vi "Fetch.vi"(8 "error in (no error)":errorcluster, 10 "Message in":refnum<class "FetchMessage.lvclass">, 11 "BMC in":refnum<class "BMC.lvclass">) -> (0 "error out":errorcluster, 3 "BMC out":refnum<class "BMC.lvclass">)   [LabVIEW 2012, in "BMC.lvclass"]
doc: "The fetch method processes the command 'fetch'. \n\nThe command 'fetch' is used for receiving various forms of data."
uses:
  BMC.lvclass
  <vilib>/Distrio/Murmex/FetchMessage/FetchMessage.lvclass
  <vilib>/Distrio/Murmex/Murmex/Murmex.lvclass
  BMC.lvclass/BMC.ctl
panel:
  out "actuator":dbl
  out "1x160 voltage array":dbl[](array[numeric])
  # "This method is called when the FETCH\ntrigger is sent. \n\nOverride this method when your component needs to\nrespond to this trigger. \n\nCall parent for proper implementation"
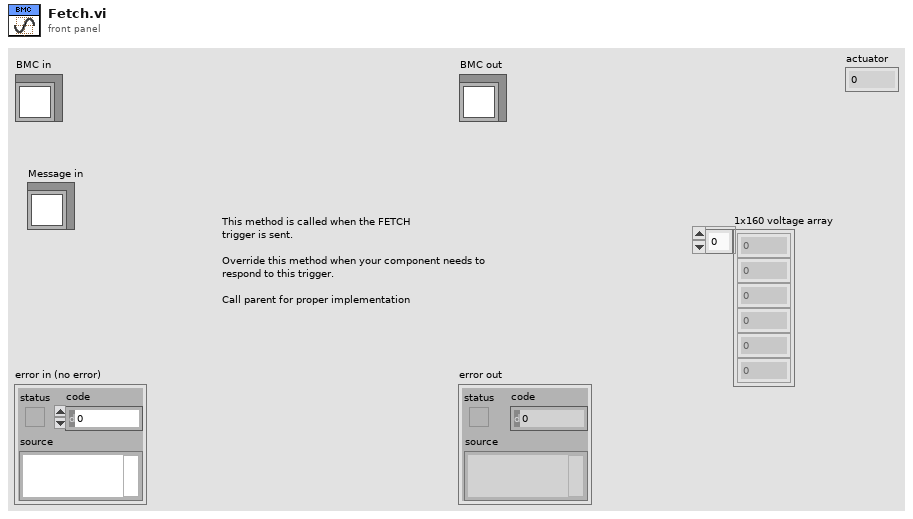
[diagram p1: front panel]
types:
  T1 = typedef "Murmex.lvlib/FetchMessage.lvclass/Channel data cluster.ctl" = cluster{"channel id":i32, "data UInt8":u8[], "data type":T2, "dimensions":i32[], "physical units":T3[], "waveform dt":dbl, "waveform":T4}
  T2 = typedef "Murmex.lvlib/Murmex.lvclass/data_type_enum.ctl" = enum16{"Float128", "Float64", "Float32", "Int64", "Int32", "Int16", "Int8", "UInt64", "UInt32", "UInt16", "UInt8", "Boolean", "String"}
  T3 = typedef "Physical Units__ogtk.ctl" = cluster{"Base Units":enum16{"radian", "steradian", "second", "meter", "kilogram", "ampere", "kelvin", "mole", "candela"}, "Exponent":i16}
  T4 = typedef "Murmex.lvlib/Murmex.lvclass/waveform_type_enum.ctl" = enum16{"no waveform", "analog", "digital"}
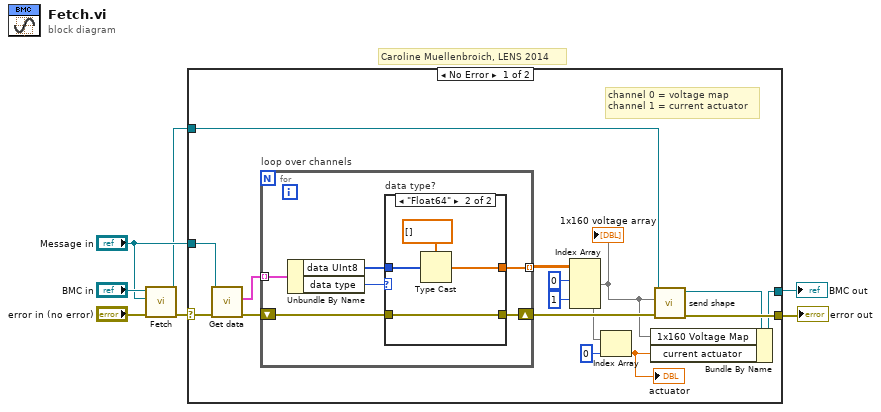
[diagram p0: block diagram]
diagram:
  # "Caroline Muellenbroich, LENS 2014"
  n1 = call-parent "Fetch.vi"("error in (no error)"="error in (no error)", "Message in"="Message in", "Murmex in"="BMC in") -> ("error out"=w4:errorcluster, "Murmex out"=w3:refnum<class "BMC.lvclass">)  [unwired: 7 in]
  n2 = case shown="No Error" w4 {
    selector: w4 -> [w22 w35]
    tunnel: "Message in" -> [w23 _]
    tunnel: w3 -> [w17 w36]
    tunnel: [w10 w36] -> w2
    tunnel: [w18 w35] -> w1
    frame No Error {
      # "channel 0 = voltage map\nchannel 1 = current actuator"
      n3 = call <vilib>:"Get data.vi"("error in (no error)"=w22, "FetchMessage.lvclass"=w23) -> ("error out"=w21:errorcluster, "data (channels)"=w20:T1[])  [unwired: 7 in, 1 out]
      n4 = for "loop over channels" {
        tunnel: w20 -> [w27] mode=indexing
        shift-right: [w25] -> w19
        shift-left: w21 -> [w26]
        tunnel: [w24] -> w16 mode=indexing
        n5 = Unbundle By Name(w27) -> ("data UInt8"=w29:u8[], "data type"=w28:T2)
        n6 = case "data type?" shown="\"Float64\"" w28 {
          tunnel: w29 -> [_ w34]
          tunnel: [_ w33] -> w24
          tunnel: w26 -> [w30 w31]
          tunnel: [w30 w31] -> w25
          frame Default {
          }
          frame "Float64" {
            n7 = Type Cast(type=dbl[] [] ("run time Cluster.1x160 Voltage Map"), x=w34) -> (*(type *) &x=w33:dbl[])
          }
        }
      }
      n8 = Index Array(array=w16, index (row) #1=0 ("index (row)"), index (row) #2=1 ("index (row)")) -> (element #1=w8:dbl[], element #2=w13:dbl[])  [unwired: 2 in]
      "1x160 voltage array" <- w8
      n9 = Index Array(array=w13, index=0) -> (element=w9:dbl)
      "actuator" <- w9
      n10 = call-dynamic "send shape.vi"("error in (no error)"=w19, "1x160 Voltage Map"=w8, "BMC in"=w17) -> ("error out"=w18:errorcluster, "BMC out"=w11:refnum<class "BMC.lvclass">)  [unwired: 7 in]
      n11 = Bundle By Name(cluster=w11, "1x160 Voltage Map"=w8, "current actuator"=w9) -> (w10:refnum<class "BMC.lvclass">)
    }
    frame Error {
    }
  }
  "error out" <- w1
  "BMC out" <- w2
